vi "A170316-11-Login.vi"() -> ()   [LabVIEW 2020]
uses:
  Database/Global1.vi
  <vilib>/addons/database/Connection.llb/DB Tools Open Connec (String).vi
  <vilib>/addons/database/Connection.llb/Conn Execute.vi
  <vilib>/addons/database/Recordset.llb/Rec Fetch Recordset Data (R).vi
  <vilib>/addons/database/NI_Database_API.lvlib
  <vilib>/addons/database/Recordset.llb/Rec Destroy - Connection.vi
panel:
  in  "登陆":bool
  in  "密   码":string
  out "数据库连接成功":bool
  in  "联机模式":enum16{"单机", "联网"}(ring)
  in  "用户名":string
  # "数据库状态"
  # "电机ECU装配"
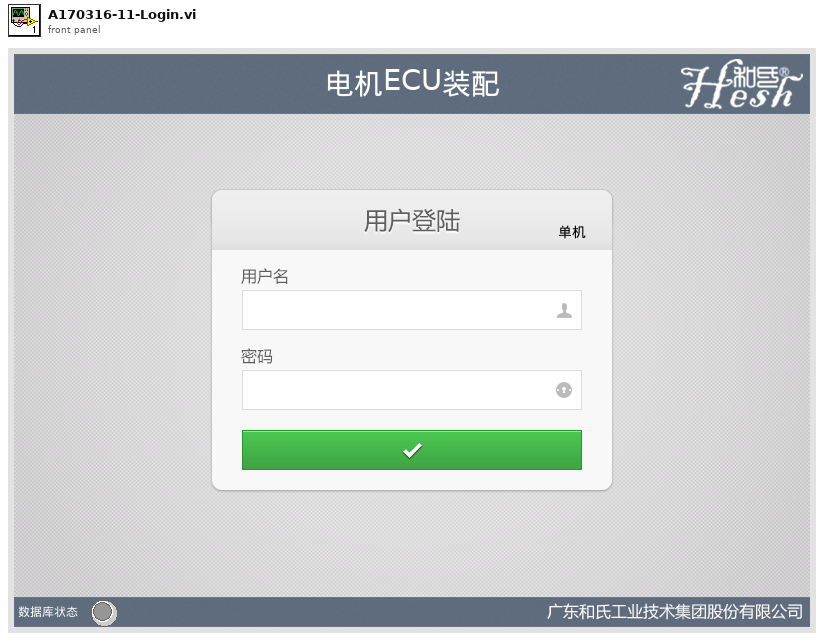
[diagram p1: front panel]
types:
  T1 = enum8{"Enabled", "Disabled", "Disabled and Grayed Out"}
  T2 = enum32{"Invalid", "Standard", "Closed", "Hidden", "Minimized", "Maximized"}
  T3 = cluster{"data[0]":string, "data[1]":string, "data[2]":string, "data[3]":string}
  T4 = typedef "NI_Database_API.lvlib/Conn ObjectReference.ctl" = refnum<k1>
  T5 = typedef "NI_Database_API.lvlib/Rec ObjectReference.ctl" = refnum<k1>
  T6 = typedef "eventvkey.ctl" = enum16{"ASCII", "Enter", "Return", "Shift", "Ctrl", "Alt", "Cmd", "Opt", "Caps", "NumLock", "Clear", "Break", "Up", "Down", "Left", "Right", "Insert", "Delete", "Home", "End", "PageUp", "PageDown", "Escape", "Help", "Pause", "ScrollLock", "F1", "F2", "F3", "F4", "F5", "F6", "F7", "F8", "F9", "F10", "F11", "F12", "F13", "F14", "F15", "F16", "F17", "F18", "F19", "F20", "F21", "F22", "F23", "F24", "Play", "VolumeUp", "VolumeDown", "Mute", "Two Byte Char"}
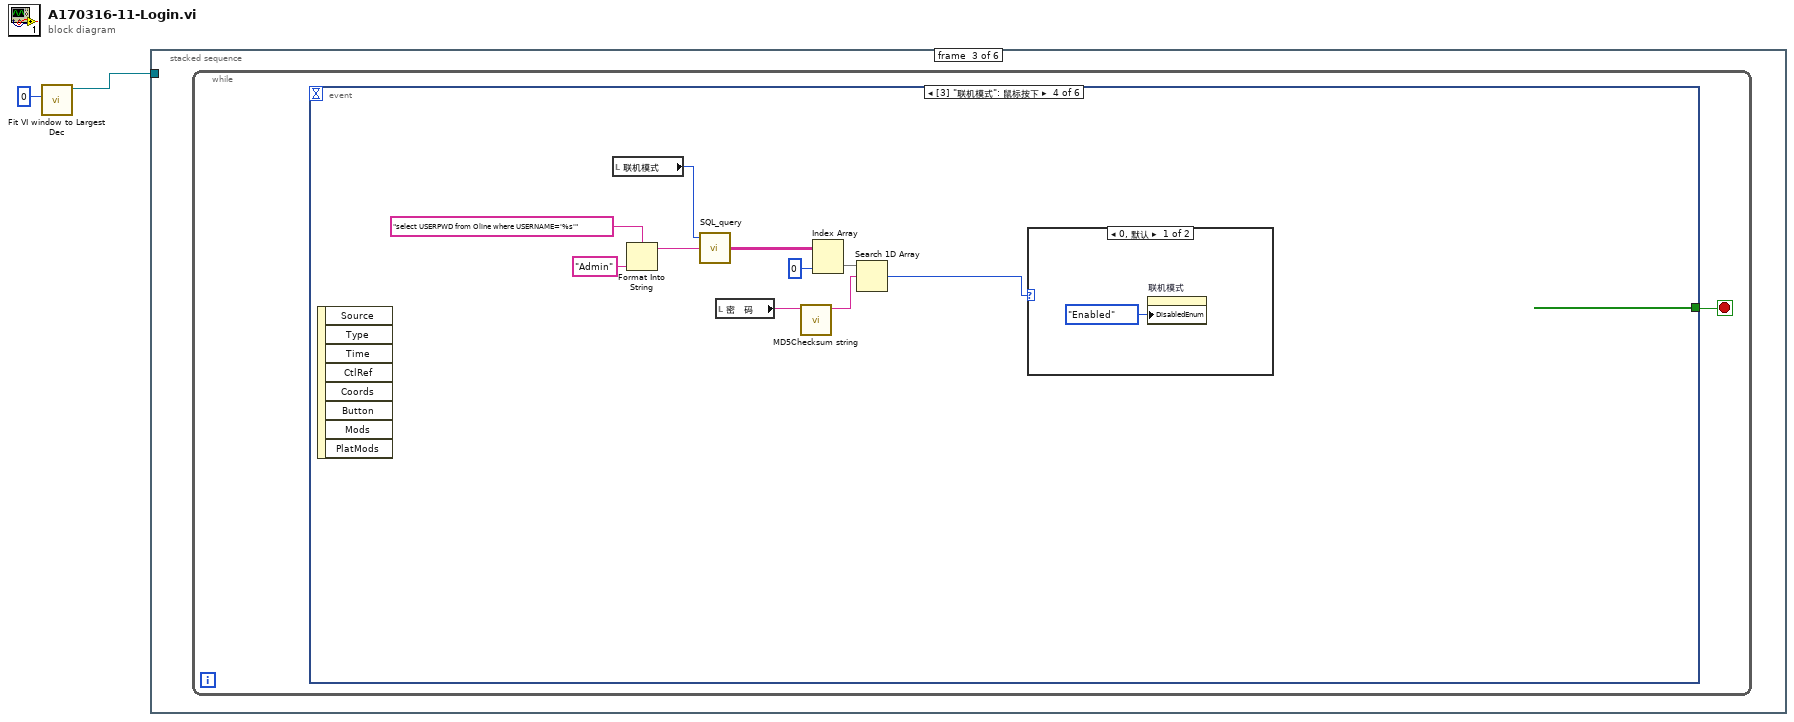
[diagram p0: block diagram]
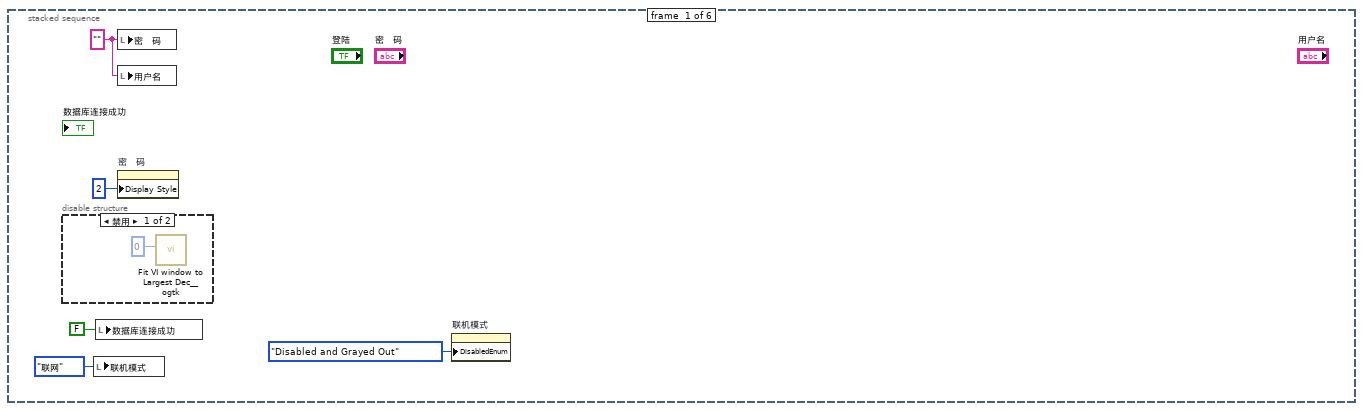
[diagram p2: hidden frame]
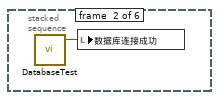
[diagram p4: hidden frame]
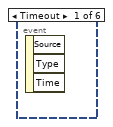
[diagram p5: hidden frame]
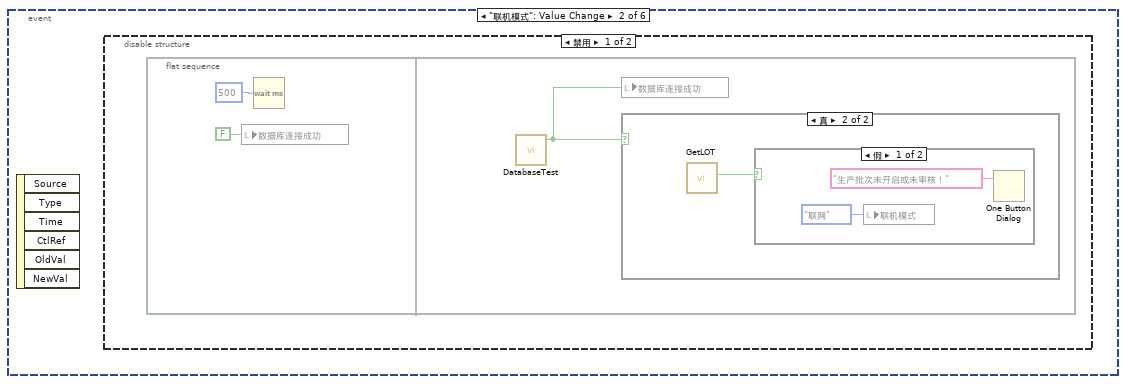
[diagram p6: hidden frame]
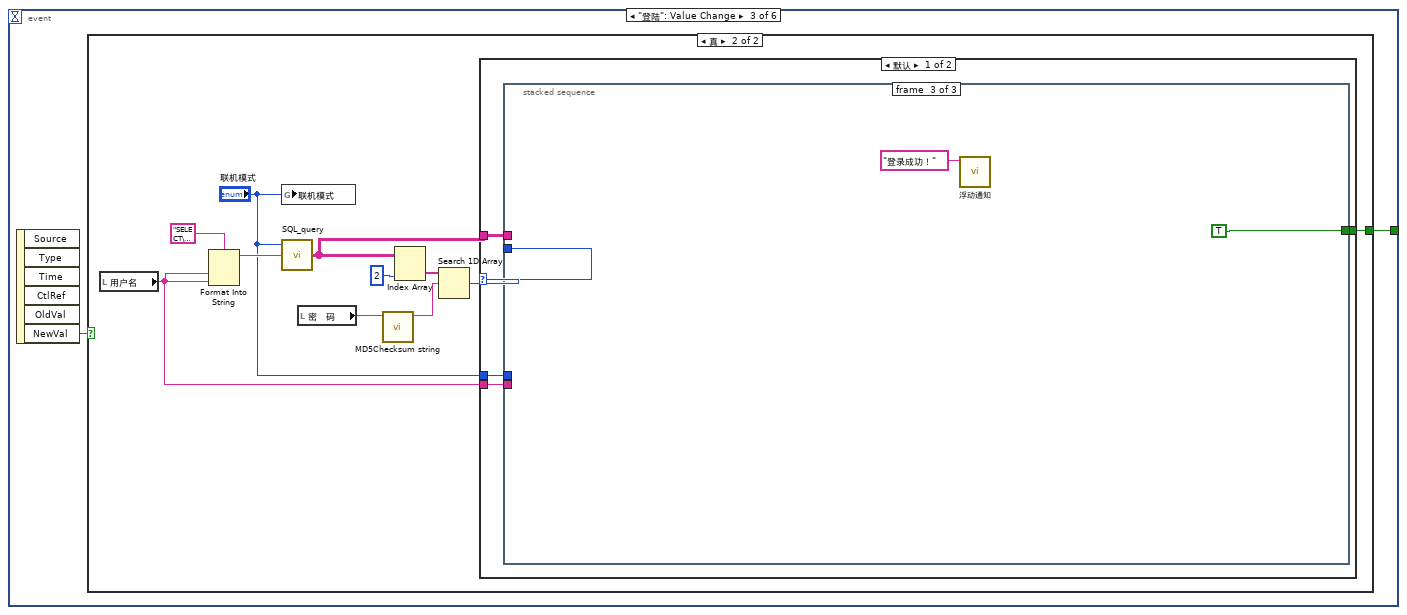
[diagram p10: hidden frame]
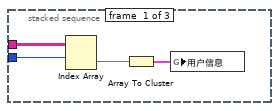
[diagram p12: hidden frame]
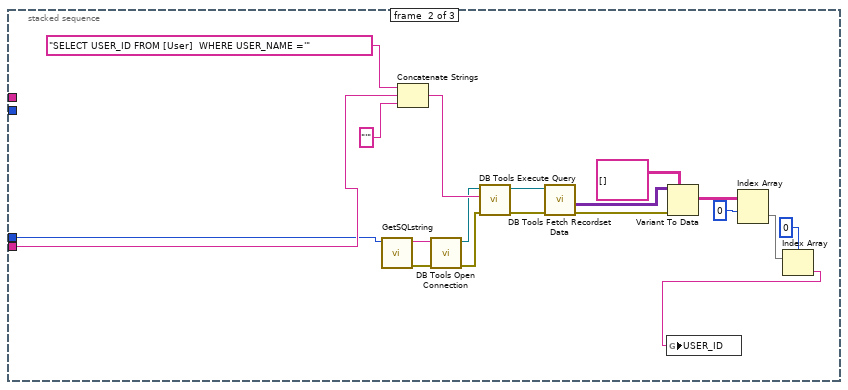
[diagram p13: hidden frame]
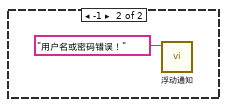
[diagram p14: hidden frame]
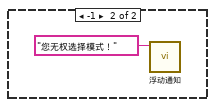
[diagram p15: hidden frame]
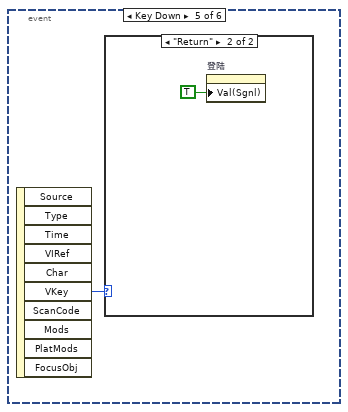
[diagram p16: hidden frame]
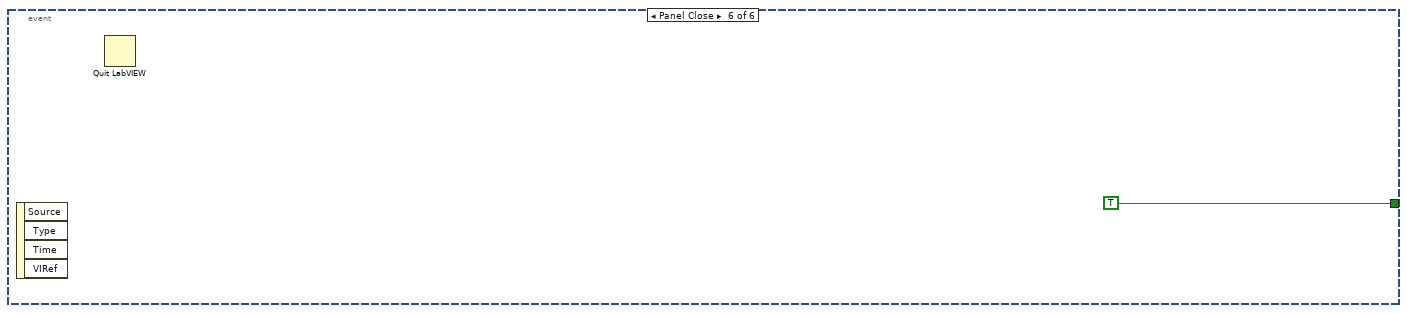
[diagram p18: hidden frame]
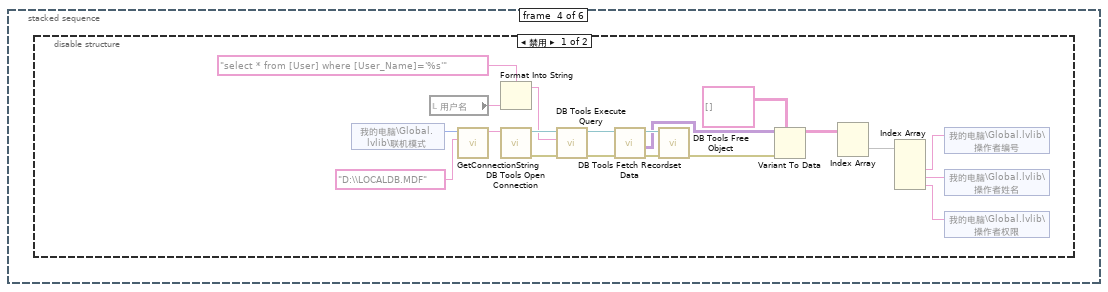
[diagram p19: hidden frame]
diagram:
  n1 = call "Fit VI window to Largest Dec.vi"("border spacing (2 px)"=0) -> ("dup VI Ref"=w1:refnum<vi>)  [unwired: 5 in, 1 out]
  n2 = stacked-sequence {
    tunnel: w1 -> [_ _ _ _ _ _]
    frame #0 {
      w6 = ""
      n3 = disable-structure shown="禁用" {
        frame Disabled {
          n4 = call <userlib>:"Fit VI window to Largest Dec__ogtk.vi"("border spacing (2 px)"=0) -> ()  [unwired: 5 in, 2 out]
        }
        frame Enabled {
        }
      }
      n5 = local write "联机模式"(enum16{"单机", "联网"}."联网" ("联机模式")) -> ()
      n6 = local write "数据库连接成功"(FALSE ("数据库连接成功")) -> ()
      n7 = local write "密   码"(w6) -> ()
      n8 = local write "用户名"(w6) -> ()
      n9 = property on="密   码" class="Str"("Display Style"=u32 2 ("显示样式")) -> ()  [unwired: 2 in, 2 out]
      n10 = property on="联机模式" class="Enum (严格)"("DisabledEnum"=T1."Disabled and Grayed Out" ("禁用")) -> ()  [unwired: 2 in, 2 out]
    }
    frame #1 {
      n11 = call "DatabaseTest.vi"() -> ("数据库连接成功"=w9:bool)  [unwired: 4 in, 1 out]
      n12 = local write "数据库连接成功"(w9) -> ()
    }
    frame #2 {
      n13 = while {
        stop <- w10 stop-if-true
        n14 = event shown="[3] \"联机模式\": 鼠标按下" {
          selector: _ -> [_ _ _ _ _ _]
          dyn-events: _ -> [_ _ _ _ _ _]
          timeout: _ -> [_ _ _ _ _ _]
          tunnel: [_ _ w17 _ _ TRUE] -> w10
          event Timeout {
            n15 = event-data() -> ()  [unwired: 1 in, 3 out]
          }
          event "联机模式": Value Change {
            n16 = event-data() -> ()  [unwired: 1 in, 6 out]
            n17 = disable-structure shown="禁用" {
              frame Disabled {
                n18 = flat-sequence {
                  frame #0 {
                    n19 = local write "数据库连接成功"(FALSE ("数据库连接成功")) -> ()
                    n20 = Wait (ms)(milliseconds to wait=u32 500 ("等待时间（毫秒）")) -> ()  [unwired: 1 out]
                  }
                  frame #1 {
                    n21 = call "DatabaseTest.vi"() -> ("数据库连接成功"=w13:bool)  [unwired: 4 in, 1 out]
                    n22 = local write "数据库连接成功"(w13) -> ()
                    n23 = case shown="真" w13 {
                      frame False {
                      }
                      frame True {
                        n24 = call "GetLOT.vi"() -> ("生产批次有效"=w14:bool)  [unwired: 9 in, 2 out]
                        n25 = case shown="假" w14 {
                          frame False {
                            n26 = local write "联机模式"(enum16{"单机", "联网"}."联网" ("联机模式")) -> ()
                            n27 = One Button Dialog(message="生产批次未开启或未审核！" ("消息")) -> ()  [unwired: 1 in, 1 out]
                          }
                          frame True {
                          }
                        }
                      }
                    }
                  }
                }
              }
              frame Enabled {
              }
            }
          }
          event "登陆": Value Change {
            n28 = event-data() -> ("NewVal"=w18:bool)  [unwired: 1 in, 5 out]
            n29 = case shown="真" w18 {
              tunnel: [_ w21] -> w17
              frame False {
              }
              frame True {
                n30 = local read "用户名"() -> (w20:string)
                n31 = Format Into String(format string="SELECT\ndbo.[User].USER_EMPLOYEE_ID,\ndbo.[User].USER_NAME,\ndbo.[User].USER_PASSWD,\ndbo.[User].USER_PERMIT\n\nFROM\ndbo.[User]\nWHERE\ndbo.[User].USER_NAME = '%s' \nOR\ndbo.[User].USER_EMPLOYEE_ID = '%s'\n" ("格式字符串"), w20, w20) -> (resulting string=w27:string)  [unwired: 2 in, 1 out]
                n32 = global write "Global1.vi" "联机模式"("联机模式") -> ()
                n33 = call "SQL_query.vi"("SQL query"=w27, "联机模式"="联机模式") -> ("data"=w22:string[][])  [unwired: 1 in, 2 out]
                n34 = local read "密   码"() -> (w29:string)
                n35 = call <vilib>:"MD5Checksum string.vi"("Message String"=w29) -> ("MD5 message-digest"=w23:string)  [unwired: 10 in]
                n36 = Index Array(array=w22, index (col)=2 ("禁用的索引 (列)")) -> (element=w26:string[])  [unwired: 1 in]
                n37 = Search 1D Array(1D array=w26, element=w23) -> (index of element=w24:i32)  [unwired: 1 in]
                n38 = case shown="默认" w24 {
                  selector: w24 -> [w34 _]
                  tunnel: w22 -> [w33 _]
                  tunnel: [w32 _] -> w21
                  tunnel: w20 -> [w31 _]
                  tunnel: "联机模式" -> [w30 _]
                  frame Default {
                    n39 = stacked-sequence {
                      tunnel: w34 -> [w35 _ _]
                      tunnel: w33 -> [w37 _ _]
                      tunnel: [_ _ TRUE] -> w32
                      tunnel: w31 -> [_ w41 _]
                      tunnel: w30 -> [_ w40 _]
                      frame #0 {
                        n40 = Index Array(array=w37, index (row)=w35) -> (element=w36:string[])  [unwired: 1 in]
                        n41 = Array To Cluster(array=w36) -> (cluster=w38:T3)
                        n42 = global write "Global1.vi" "用户信息"(w38) -> ()
                      }
                      frame #1 {
                        n43 = call "GetSQLstring.vi"("联机模式"=w40) -> ("错误输出"=w56:errorcluster, "连接字符串"=w57:string)  [unwired: 9 in]
                        n44 = Concatenate Strings("SELECT USER_ID FROM [User]  WHERE USER_NAME ='" ("字符串"), w41, "'" ("字符串")) -> (w55:string)
                        n45 = call-poly <vilib>:"DB Tools Open Connection.vi"("error in (no error)"=w56, "connection information"=w57) -> ("error out"=w49:errorcluster, "connection reference"=w50:T4)  [unwired: 6 in]
                        n46 = call-poly <vilib>:"DB Tools Execute Query.vi"("error in (no error)"=w49, "SQL query"=w55, "connection reference"=w50) -> ("error out"=w53:errorcluster, "recordset reference"=w54:T5)  [unwired: 5 in]
                        n47 = call-poly <vilib>:"DB Tools Fetch Recordset Data.vi"("error in (no error)"=w53, "recordset reference"=w54) -> ("error out"=w47:errorcluster, "recordset data"=w52:variant[][])  [unwired: 3 in, 1 out]
                        n48 = Variant To Data(error in=w47, type=string[][] [], Variant=w52) -> (data=w46:string[][])  [unwired: 1 out]
                        n49 = Index Array(array=w46, index (row)=0 ("索引 (行)")) -> (element=w44:string[])  [unwired: 1 in]
                        n50 = Index Array(array=w44, index=0 ("索引 (行)")) -> (element=w39:string)
                        n51 = global write "Global1.vi" "USER_ID"(w39) -> ()
                      }
                      frame #2 {
                        n52 = call "浮动通知.vi"("通知内容"="登录成功！") -> ()  [unwired: 11 in]
                      }
                    }
                  }
                  frame -1 {
                    n53 = call "浮动通知.vi"("通知内容"="用户名或密码错误！") -> ()  [unwired: 11 in]
                  }
                }
              }
            }
          }
          event "联机模式": Mouse Down {
            n54 = event-data() -> ()  [unwired: 1 in, 8 out]
            n55 = local read "联机模式"() -> (w63:enum16{"单机", "联网"})
            n56 = Format Into String(format string="select USERPWD from Oline where USERNAME='%s'" ("格式字符串"), "Admin" ("输入 1")) -> (resulting string=w69:string)  [unwired: 2 in, 1 out]
            n57 = call "SQL_query.vi"("SQL query"=w69, "联机模式"=w63) -> ("data"=w66:string[][])  [unwired: 1 in, 2 out]
            n58 = local read "密   码"() -> (w70:string)
            n59 = call <vilib>:"MD5Checksum string.vi"("Message String"=w70) -> ("MD5 message-digest"=w67:string)  [unwired: 10 in]
            n60 = Index Array(array=w66, index (col)=0 ("禁用的索引 (列)")) -> (element=w68:string[])  [unwired: 1 in]
            n61 = Search 1D Array(1D array=w68, element=w67) -> (index of element=w62:i32)  [unwired: 1 in]
            n62 = case shown="0, 默认" w62 {
              frame 0, Default {
                n63 = property on="联机模式" class="Enum (严格)"("DisabledEnum"=T1."Enabled" ("禁用")) -> ()  [unwired: 2 in, 2 out]
              }
              frame -1 {
                n64 = call "浮动通知.vi"("通知内容"="您无权选择模式！") -> ()  [unwired: 11 in]
              }
            }
          }
          event Key Down {
            n65 = event-data() -> ("VKey"=w73:T6)  [unwired: 1 in, 9 out]
            n66 = case shown="\"Return\"" w73 {
              frame "ASCII", Default {
              }
              frame "Return" {
                n67 = property on="登陆" class="Bool (严格)"("Val(Sgnl)"=TRUE ("值(信号)")) -> ()  [unwired: 2 in, 2 out]
              }
            }
          }
          event Panel Close {
            n68 = event-data() -> ()  [unwired: 1 in, 4 out]
            n69 = Quit LabVIEW() -> ()  [unwired: 1 in]
          }
        }
      }
    }
    frame #3 {
      n70 = disable-structure shown="禁用" {
        frame Disabled {
          n71 = shared-variable "我的电脑\\Global.lvlib\\联机模式"() -> (w76:i16)  [unwired: 1 in, 1 out]
          n72 = local read "用户名"() -> (w78:string)
          n73 = call "GetConnectionString.vi"("Database Name"="D:\\LOCALDB.MDF", "连接模式"=w76) -> ("连接字符串"=w94:string)  [unwired: 4 in, 1 out]
          n74 = Format Into String(format string="select * from [User] where [User_Name]='%s'", w78) -> (resulting string=w77:string)  [unwired: 2 in, 1 out]
          n75 = call-poly <vilib>:"DB Tools Open Connection.vi"("connection information"=w94) -> ("error out"=w93:errorcluster, "connection reference"=w92:T4)  [unwired: 7 in]
          n76 = call-poly <vilib>:"DB Tools Execute Query.vi"("error in (no error)"=w93, "SQL query"=w77, "connection reference"=w92) -> ("error out"=w89:errorcluster, "recordset reference"=w91:T5)  [unwired: 5 in]
          n77 = call-poly <vilib>:"DB Tools Fetch Recordset Data.vi"("error in (no error)"=w89, "recordset reference"=w91) -> ("error out"=w88:errorcluster, "recordset data"=w86:variant[][], "recordset reference out"=w90:T5)  [unwired: 3 in]
          n78 = call-poly <vilib>:"DB Tools Free Object.vi"("error in (no error)"=w88, "recordset reference"=w90) -> ("error out"=w87:errorcluster)  [unwired: 8 in, 1 out]
          n79 = Variant To Data(error in=w87, type=string[][] [], Variant=w86) -> (data=w84:string[][])  [unwired: 1 out]
          n80 = Index Array(array=w84) -> (element=w83:string[])  [unwired: 2 in]
          n81 = Index Array(array=w83) -> (element #2=w80:string, element #3=w81:string, element #4=w82:string)  [unwired: 4 in, 1 out]
          n82 = shared-variable "我的电脑\\Global.lvlib\\操作者编号"(w80) -> ()  [unwired: 1 in, 1 out]
          n83 = shared-variable "我的电脑\\Global.lvlib\\操作者姓名"(w81) -> ()  [unwired: 1 in, 1 out]
          n84 = shared-variable "我的电脑\\Global.lvlib\\操作者权限"(w82) -> ()  [unwired: 1 in, 1 out]
        }
        frame Enabled {
        }
      }
    }
    frame #4 {
      n85 = vi-ref "A170316-11-Main-large.vi"() -> (w97:refnum<vi>)
      n86 = call "CallVI.vi"("VI引用"=w97, "状态"=T2."Maximized") -> ()  [unwired: 11 in, 3 out]
    }
    frame #5 {
      n87 = control-ref of="本VI"() -> (w98:refnum<vi>)
      n88 = invoke class="VI" method="FP.Close"(reference=w98) -> (reference out=w99:refnum<vi>, error out=w100:errorcluster)  [unwired: 2 in, 1 out]
      n89 = Close Reference(reference=w99, error in (no error)=w100) -> ()  [unwired: 1 out]
    }
  }
